vi "Read ADC.vi"(8 "error in (no error)":errorcluster, 10 "ADC Channel":dbl, 11 "object in":refnum<class "Arduino.lvclass">) -> (0 "error out":errorcluster, 3 "object out":refnum<class "Arduino.lvclass">)   [LabVIEW 2020, in "Arduino.lvclass"]
doc: "Read ADC es el vi donde se manda al microcontrolador los datos del canal analogico que se desea leer"
uses:
  Arduino.lvclass
  Arduino.lvclass/Arduino.ctl
  7aab8b69-ef43-4b20-97e2-7b7ea187d284.vi
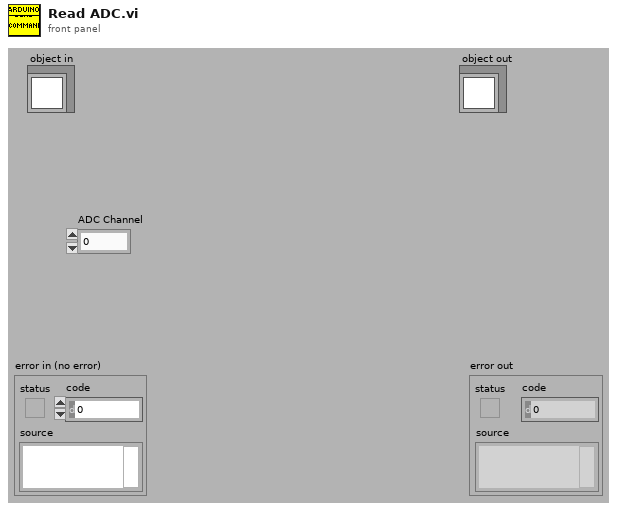
[diagram p1: front panel]
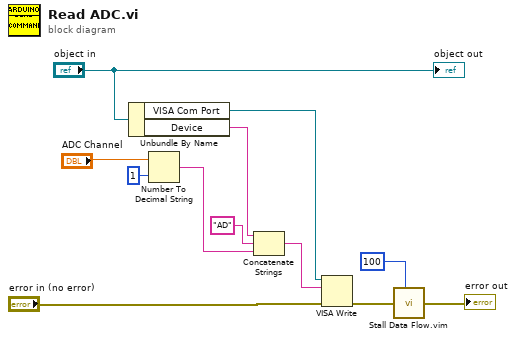
[diagram p0: block diagram]
diagram:
  n1 = Unbundle By Name("object in") -> ("VISA Com Port"=w11:refnum<visa-resource-name>, "Device"=w9:string)
  n2 = Number To Decimal String(number="ADC Channel", width (-)=i16 1) -> (decimal integer string=w8:string)
  n3 = Concatenate Strings(w9, "AD" ("string"), w8) -> (w10:string)
  n4 = VISA Write(VISA resource name=w11, write buffer=w10, error in (no error)="error in (no error)") -> (error out=w12:errorcluster)  [unwired: 2 out]
  n5 = call "Stall Data Flow.vim"("value in"=w12, "milliseconds to wait"=u32 100) -> ("value out"=→"error out":errorcluster)  [unwired: 1 out]
  "object out" <- "object in"
